vi "FindEqualName(SubVI).vi"(1 "Name":string, 2 "Strings And Values[]":cluster{"String":string, "Value":string}[](array[cluster])) -> (0 "Does the array contain this name?":bool)   [LabVIEW 2018]
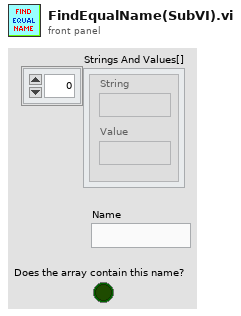
[diagram p1: front panel]
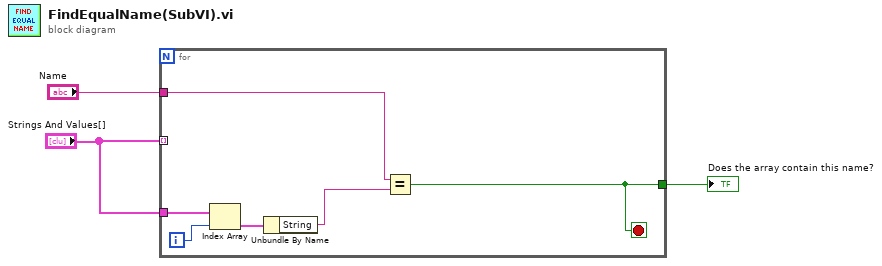
[diagram p0: block diagram]
diagram:
  n1 = for {
    tunnel: "Strings And Values[]" -> [_] mode=indexing
    tunnel: "Strings And Values[]" -> [w9]
    tunnel: "Name" -> [w6]
    tunnel: [w4] -> w1
    i -> [w8]
    stop <- w4 stop-if-true
    n2 = Index Array(array=w9, index=w8) -> (element=w7:cluster{"String":string, "Value":string})
    n3 = Unbundle By Name(w7) -> ("String"=w5:string)
    n4 = Equal?(x=w6, y=w5) -> (x = y?=w4:bool)
  }
  "Does the array contain this name?" <- w1
